vi "ActivDesactivCtrl.vi"(4 "error in (no error)":errorcluster, 6 "Disabled":T1(ring), 7 "Cluster":T2) -> (0 "error out":errorcluster)   [LabVIEW 2017]
uses:
  DefDeType/ClusterRefCtrl.ctl
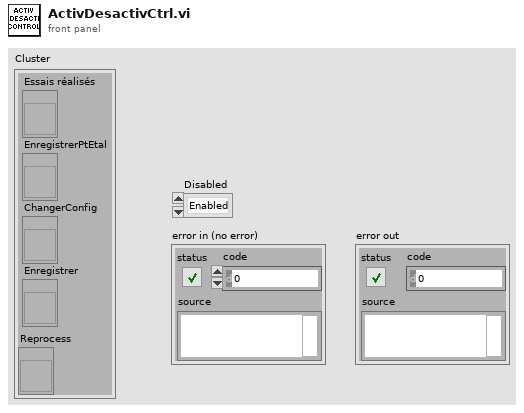
[diagram p1: front panel]
types:
  T1 = enum8{"Enabled", "Disabled", "Disabled and Grayed Out"}
  T2 = typedef "ClusterRefCtrl.ctl" = cluster{"Essais réalisés":refnum<vi>, "EnregistrerPtEtal":refnum<vi>, "ChangerConfig":refnum<vi>, "Enregistrer":refnum<vi>, "Reprocess":refnum<vi>}
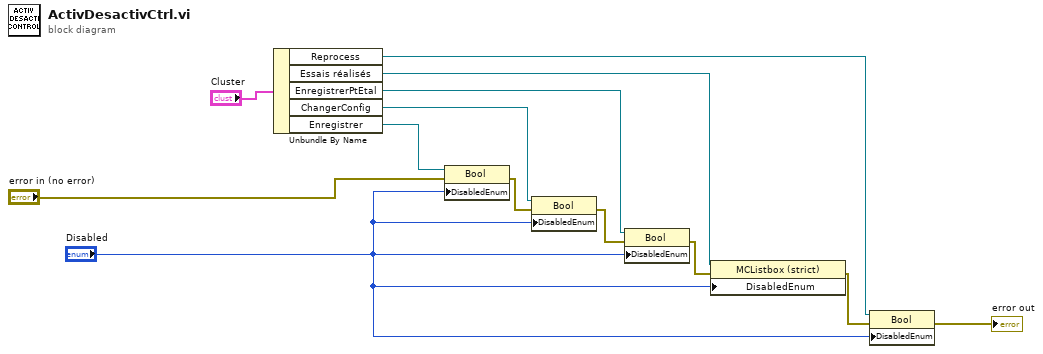
[diagram p0: block diagram]
diagram:
  n1 = Unbundle By Name("Cluster") -> ("Reprocess"=w2:refnum<vi>, "Essais réalisés"=w10:refnum<vi>, "EnregistrerPtEtal"=w11:refnum<vi>, "ChangerConfig"=w12:refnum<vi>, "Enregistrer"=w13:refnum<vi>)
  n2 = property class="Bool"(reference=w13, error in="error in (no error)", "DisabledEnum"="Disabled") -> (error out=w6:errorcluster)  [unwired: 1 out]
  n3 = property class="Bool"(reference=w12, error in=w6, "DisabledEnum"="Disabled") -> (error out=w7:errorcluster)  [unwired: 1 out]
  n4 = property class="Bool"(reference=w11, error in=w7, "DisabledEnum"="Disabled") -> (error out=w8:errorcluster)  [unwired: 1 out]
  n5 = property class="MCListbox (strict)"(reference=w10, error in=w8, "DisabledEnum"="Disabled") -> (error out=w4:errorcluster)  [unwired: 1 out]
  n6 = property class="Bool"(reference=w2, error in=w4, "DisabledEnum"="Disabled") -> (error out=→"error out":errorcluster)  [unwired: 1 out]
